vi "test_firebase_db.vi"() -> ()   [LabVIEW 2016]
uses:
  <vilib>/httpClient/PUTBuffer.vi
  <vilib>/httpClient/LabVIEWHTTPClient.lvlib
panel:
  out "값":cluster{"name":string, "val":dbl, "onoff":bool}
  in  "R/W":bool
  in  "onoff":bool
  in  "val":dbl
  in  "name":string
  out "연결된 문자열":string="{\"test\":0.90723410097909862}"
  out "body":string="{\"test\":0.9072341009790986}" caption="본문"
  out "headers":string="HTTP/1.1 100 Continue\r\n\r\nHTTP/1.1 200 OK\r\nServer: nginx\r\nDate: Tue, 24 Apr 2018 08:22:22 GMT\r\nContent-Type: application/json; charset=utf-8\r\nContent-Length: 27\r\nConnection: keep-alive\r\nAccess-Control-Allow-Origin: *\r\nCache-Control: no-cache\r\nStrict-Transport-Security: max-age=31556926; includeSubDomains; preload\r\n\r\n" caption="헤더"
  out "error out":errorcluster caption="에러 출력"
  in  "정지":bool
  in  "Firebase url":string="https://motlab-81406.firebaseio.com/.json"
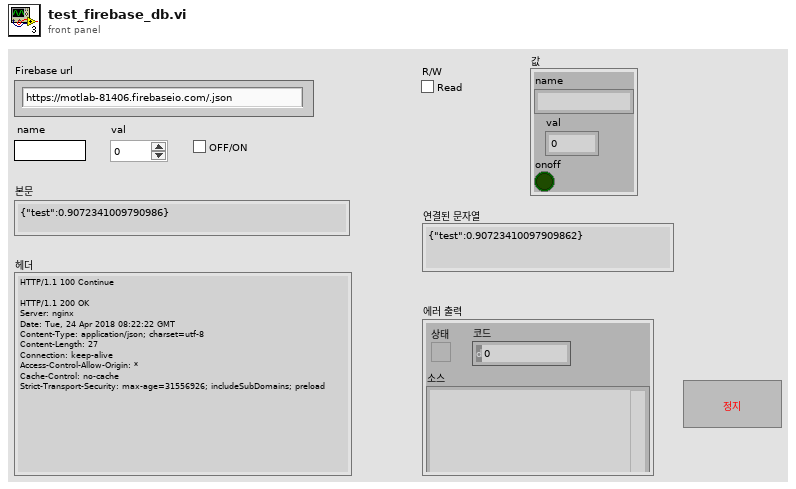
[diagram p1: front panel]
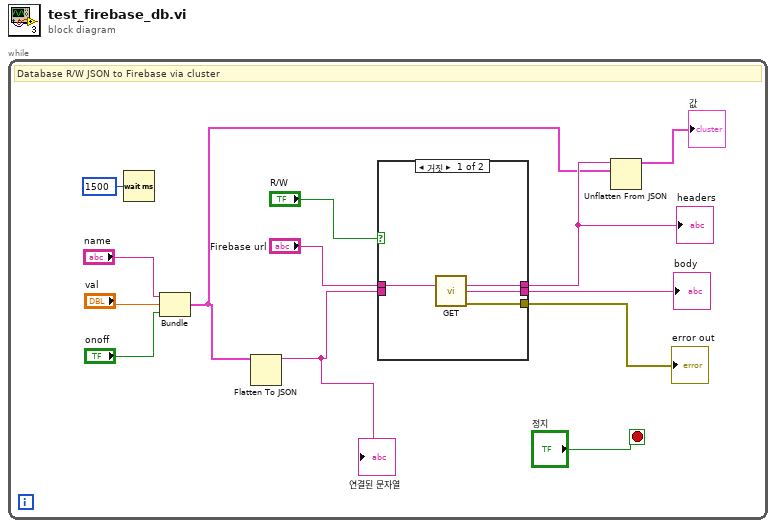
[diagram p0: block diagram]
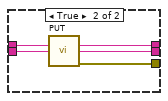
[diagram p2: hidden frame]
diagram:
  n1 = while {
    stop <- "정지" stop-if-true
    # "Database R/W JSON to Firebase via cluster"
    n2 = Wait (ms)(milliseconds to wait=u32 1500) -> ()  [unwired: 1 out]
    n3 = Bundle("name"="name", "val"="val", "onoff"="onoff") -> (w2:cluster{"name":string, "val":dbl, "onoff":bool})  [unwired: 1 in]
    n4 = Flatten To JSON(anything=w2) -> (JSON string=w5:string)  [unwired: 2 in, 1 out]
    "연결된 문자열" <- w5
    n5 = case shown="거짓" "R/W" {
      tunnel: "Firebase url" -> [w17 w22]
      tunnel: [w16 w21] -> w10
      tunnel: [w14 w20] -> w3
      tunnel: [w15 w19] -> w9
      tunnel: w5 -> [_ w18]
      frame False {
        n6 = call <vilib>:"GET.vi"("url"=w17) -> ("headers"=w14:string, "body"=w15:string, "error out"=w16:errorcluster)  [unwired: 11 in, 1 out]
      }
      frame True {
        n7 = call-poly <vilib>:"PUT.vi"("url"=w22, "buffer"=w18) -> ("headers"=w20:string, "body"=w19:string, "error out"=w21:errorcluster)  [unwired: 10 in, 1 out]
      }
    }
    "error out" <- w10
    "headers" <- w3
    "body" <- w9
    n8 = Unflatten From JSON(JSON string=w3, type and defaults=w2) -> (value=→"값":cluster{"name":string, "val":dbl, "onoff":bool})  [unwired: 5 in, 1 out]
  }
